vi "Launch PVProxy.vi"(8 "Error In":errorcluster, 11 "CS++BaseActor in":refnum<class "CS++BaseActor.lvclass">) -> (0 "Error Out":errorcluster, 3 "CS++BaseActor out":refnum<class "CS++BaseActor.lvclass">)   [LabVIEW 2016, in "CS++BaseActor.lvlib" / "CS++BaseActor.lvclass"]
doc: "Launch PVProxy actor."
uses:
  CS++BaseActor.lvclass
  C:/Program Files (x86)/National Instruments/LabVIEW 2016/vi.lib/ActorFramework/Actor/Actor.lvclass
  CS++BaseActor.lvclass/CS++BaseActor.ctl
  <vilib>/ActorFramework/Message Enqueuer/Message Enqueuer.lvclass
  Classes/CS++BaseClasses/Factory/CS++Factory.lvclass
  <vilib>/ActorFramework/Actor/Actor.lvclass
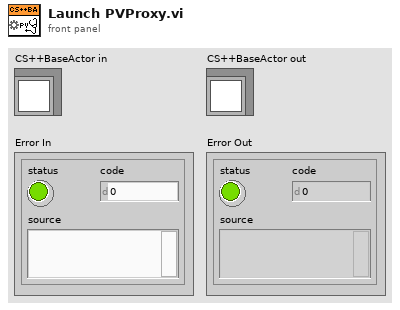
[diagram p1: front panel]
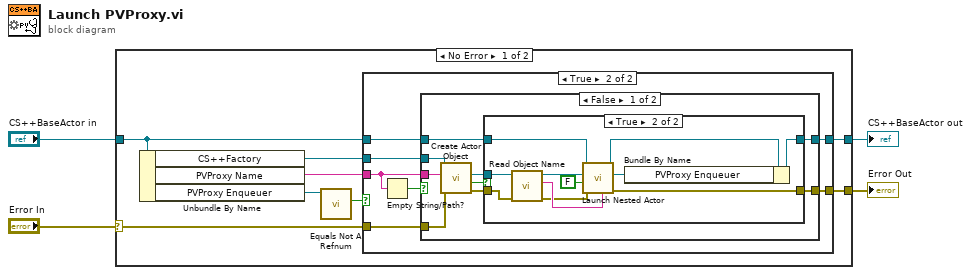
[diagram p0: block diagram]
diagram:
  n1 = case shown="No Error" "Error In" {
    selector: "Error In" -> [w11 w47]
    tunnel: [w7 w47] -> w3
    tunnel: [w8 w46] -> w1
    tunnel: "CS++BaseActor in" -> [w9 w46]
    frame No Error {
      n2 = Unbundle By Name(w9) -> ("CS++Factory"=w12:refnum<class "CS++Factory.lvclass">, "PVProxy Name"=w10:string, "PVProxy Enqueuer"=w6:refnum<class "Message Enqueuer.lvclass">)
      n3 = call <vilib>:"Equals Not A Refnum.vi"("Message Enqueuer"=w6) -> ("Not a refnum?"=w5:bool)  [unwired: 10 in]
      n4 = case shown="True" w5 {
        tunnel: w12 -> [_ w21]
        tunnel: w11 -> [w13 w20]
        tunnel: w10 -> [_ w19]
        tunnel: w9 -> [w14 w18]
        tunnel: [w14 w17] -> w8
        tunnel: [w13 w16] -> w7
        frame False {
        }
        frame True {
          n5 = Empty String/Path?(string/path=w19) -> (empty?=w15:bool)
          n6 = case shown="False" w15 {
            tunnel: w21 -> [w30 _]
            tunnel: w19 -> [w29 _]
            tunnel: w20 -> [w28 w44]
            tunnel: w18 -> [w27 w45]
            tunnel: [w24 w45] -> w17
            tunnel: [w23 w44] -> w16
            frame False {
              n7 = call "Create Actor Object.vi"("error in (no error)"=w28, "Object Name"=w29, "CS++Factory in"=w30) -> ("error out"=w26:errorcluster, "Attributes found?"=w22:bool, "CS++BaseActor"=w25:refnum<class "CS++BaseActor.lvclass">)  [unwired: 5 in, 1 out]
              n8 = case shown="True" w22 {
                tunnel: w27 -> [w32 w43]
                tunnel: w26 -> [w31 w34]
                tunnel: w25 -> [_ w37]
                tunnel: [w32 w40] -> w24
                tunnel: [w31 w39] -> w23
                frame False {
                }
                frame True {
                  n9 = call "Read Object Name.vi"("error in (no error)"=w34, "CS++BaseActor in"=w37) -> ("error out"=w33:errorcluster, "Object Name"=w35:string, "CS++BaseActor out"=w36:refnum<class "CS++BaseActor.lvclass">)  [unwired: 7 in]
                  n10 = call <vilib>:"Launch Nested Actor.vi"("Debug Alias"=w35, "error in (no error)"=w33, "Auto-stop? (T)"=FALSE, "Nested Actor"=w36, "Caller Actor in"=w43) -> ("error out"=w39:errorcluster, "Nested Actor's Enqueuer"=w41:refnum<class "Message Enqueuer.lvclass">, "Caller Actor out"=w42:refnum<class "CS++BaseActor.lvclass">)  [unwired: 4 in]
                  n11 = Bundle By Name(cluster=w42, "PVProxy Enqueuer"=w41) -> (w40:refnum<class "CS++BaseActor.lvclass">)
                }
              }
            }
            frame True {
            }
          }
        }
      }
    }
    frame Error {
    }
  }
  "Error Out" <- w3
  "CS++BaseActor out" <- w1
